vi "test-publish.vi"() -> ()   [LabVIEW 2014]
panel:
  in  "停止":bool
  out "JSON字符串 3":string
  out "JSON字符串 2":string
  out "JSON字符串":string
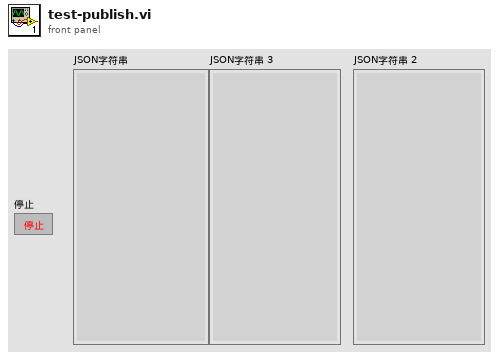
[diagram p1: front panel]
types:
  T1 = cluster{"op":string, "topic":string, "msg":cluster{"data":string}}
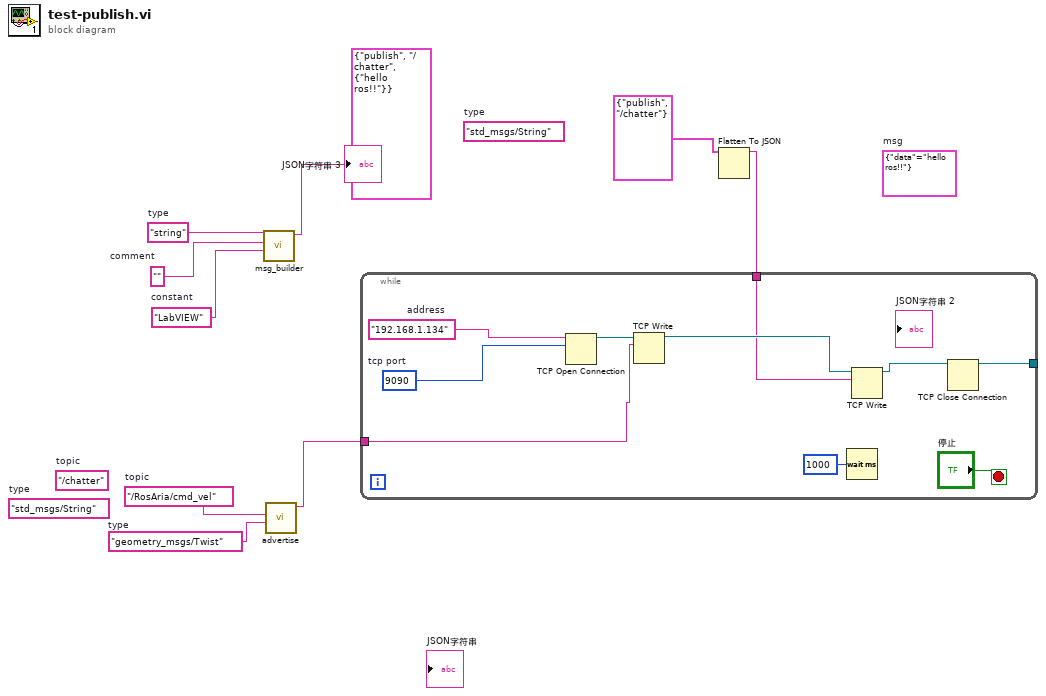
[diagram p0: block diagram]
diagram:
  (unwired) cluster{"data":string} {"data"="hello ros!!"}  # msg
  (unwired) T1 {"op"="publish", "topic"="/chatter", "msg"={"data"="hello ros!!"}}
  (unwired) "std_msgs/String"  # type
  (unwired) "/chatter"  # topic
  (unwired) "std_msgs/String"  # type
  w5 = "LabVIEW"  # constant
  w6 = ""  # comment
  w7 = "string"  # type
  w8 = "geometry_msgs/Twist"  # type
  w9 = "/RosAria/cmd_vel"  # topic
  n1 = call "msg_builder.vi"("constant"=w5, "comment"=w6, "type"=w7) -> ("msg"=→"JSON字符串 3":string)  [unwired: 8 in]
  n2 = call "advertise.vi"("type"=w8, "topic"=w9) -> ("JSON string"=w3:string)  [unwired: 9 in]
  n3 = Flatten To JSON(anything=cluster{"op":string, "topic":string} {"op"="publish", "topic"="/chatter"}) -> (JSON string=w1:string)  [unwired: 2 in, 1 out]
  n4 = while {
    tunnel: w3 -> [w14]
    tunnel: w1 -> [w12]
    tunnel: [w10] -> _
    stop <- "停止" stop-if-true
    w16 = u16 9090  # tcp port
    w15 = "192.168.1.134"  # address
    n5 = TCP Open Connection(address=w15, remote port or service name=w16) -> (connection ID=w17:refnum<k5>)  [unwired: 3 in, 1 out]
    n6 = TCP Write(connection ID=w17, data in=w14) -> (connection ID out=w13:refnum<k5>)  [unwired: 2 in, 2 out]
    n7 = Wait (ms)(milliseconds to wait=u32 1000 ("等待时间（毫秒）")) -> ()  [unwired: 1 out]
    n8 = TCP Write(connection ID=w13, data in=w12) -> (connection ID out=w11:refnum<k5>)  [unwired: 2 in, 2 out]
    n9 = TCP Close Connection(connection ID=w11) -> (connection ID out=w10:refnum<k5>)  [unwired: 2 in, 1 out]
  }
